vi "Update lvlibp Name.vi"(8 "error in (no error)":errorcluster, 10 "lvlibp name":string, 11 "NI_AB_API_PPL in":refnum<class "NI_AB_API_PPL.lvclass">) -> (0 "error out":errorcluster, 2 "Updated":bool, 3 "NI_AB_API_PPL out":refnum<class "NI_AB_API_PPL.lvclass">)   [LabVIEW 2021, in "CIF Build Actions.lvlib"]
uses:
  CIF Build Actions.lvlib
  <vilib>/AppBuilder/AB_API/PPL/NI_AB_API_PPL.lvclass
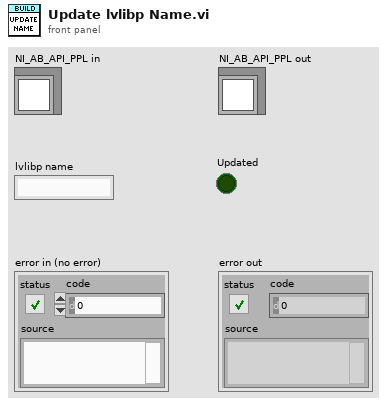
[diagram p1: front panel]
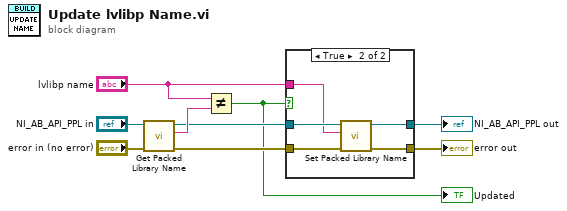
[diagram p0: block diagram]
diagram:
  n1 = call-dynamic "Get Packed Library Name.vi"("error in (no error)"="error in (no error)", "PPL in"="NI_AB_API_PPL in") -> ("error out"=w5:errorcluster, "Packed library name"=w9:string, "PPL out"=w6:refnum<class "NI_AB_API_PPL.lvclass">)  [unwired: 7 in]
  n2 = Not Equal?(x="lvlibp name", y=w9) -> (x != y?=w1:bool)
  "Updated" <- w1
  n3 = case shown="True" w1 {
    tunnel: w6 -> [w11 w16]
    tunnel: w5 -> [w10 w15]
    tunnel: [w11 w14] -> w3
    tunnel: [w10 w13] -> w2
    tunnel: "lvlibp name" -> [_ w12]
    frame False {
    }
    frame True {
      n4 = call-dynamic "Set Packed Library Name.vi"("error in (no error)"=w15, "Packed library name"=w12, "PPL in"=w16) -> ("error out"=w13:errorcluster, "PPL out"=w14:refnum<class "NI_AB_API_PPL.lvclass">)  [unwired: 7 in]
    }
  }
  "error out" <- w2
  "NI_AB_API_PPL out" <- w3
